vi "Rotation3d_Div.vi"(9 "Scalar":dbl, 11 "in Rotation3d":T1={"Q_quaternion"={"R"=1.0, "V"=[0.0, 0.0, 0.0]}}) -> (3 "out Rotation3d":T1={"Q_quaternion"={"R"=1.0, "V"=[0.0, 0.0, 0.0]}})   [LabVIEW 2019, in "Trajectory_Library.lvlib"]
doc: "Divides the current rotation by a scalar.\n\nParameters: \n- IN ROTATION3D - This ROTATION3D data structure\n- SCALAR - The value to divide the rotation by.\n\nReturns:\n - OUT ROTATION3D - THe new ROTATION3D data structure."
uses:
  TypeDef/ROTATION3D.ctl
  TypeDef/QUATERNION.ctl
  Matrix_NormF.vi
  Quaternion_New.vi
  Rotation3d_Create_Default.vi
  <vilib>/Analysis/_algsub.llb/Matrix Norm.vi
  <vilib>/Analysis/_algsub.llb/Real Matrix Norm.vi
  Quaternion_New_Default.vi
  <vilib>/Analysis/Matrix/Numeric/Conversions/Array To Matrix.vi
  <vilib>/Analysis/Matrix/Numeric/Conversions/Array To Matrix - RA.vi
  Trajectory_Library.lvlib
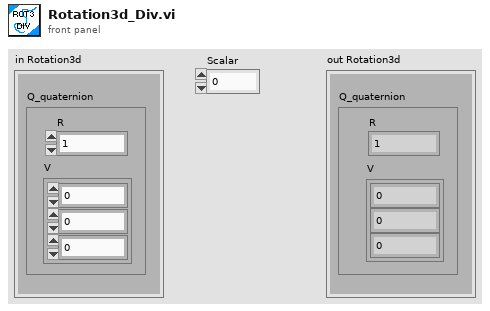
[diagram p1: front panel]
types:
  T1 = typedef "Trajectory_Library.lvlib/ROTATION3D.ctl" = cluster{"Q_quaternion":T2}
  T2 = typedef "Trajectory_Library.lvlib/QUATERNION.ctl" = cluster{"R":dbl, "V":dbl[]}
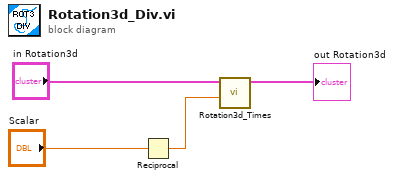
[diagram p0: block diagram]
diagram:
  n1 = Reciprocal(x="Scalar") -> (1/x=w1:dbl)
  n2 = call "Rotation3d_Times.vi"("Scalar"=w1, "in Rotation3d"="in Rotation3d") -> ("out Rotation3d"=→"out Rotation3d":T1)  [unwired: 9 in]
